vi "Constructor.vi"(8 "error in (no error)":errorcluster, 10 "Column Configuration":refnum<class "Basic Column Configuration.lvclass">, 11 "Column in":refnum<class "Column Parent.lvclass">) -> (0 "error out":errorcluster, 3 "Column out":refnum<class "Column Parent.lvclass">)   [LabVIEW 2020]
uses:
  Column Configuration/Basic Column Configuration Class/Basic Column Configuration.lvclass
  Column Parent.lvclass
  C:/Users/User/Desktop/Raman Program/Database OOP/source/Database OOP/Column Libraries/Basic Columns/Basic Columns/Column Class/Column Parent.lvclass
  C:/Users/User/Desktop/Raman Program/Database OOP/source/Database OOP/Column Libraries/Column Interface/Column Interface Class/Column Interface.lvclass
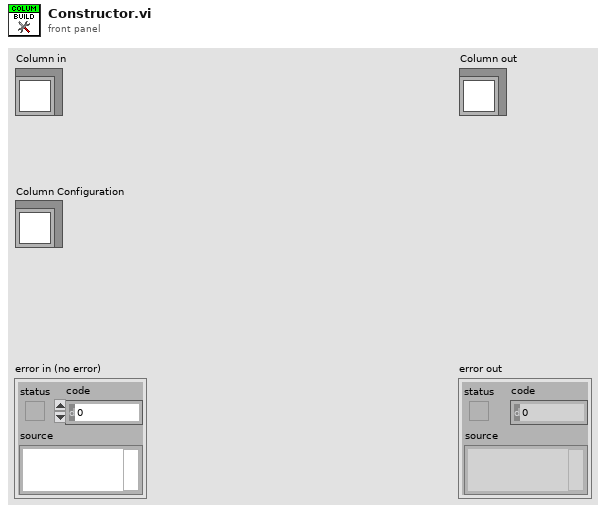
[diagram p1: front panel]
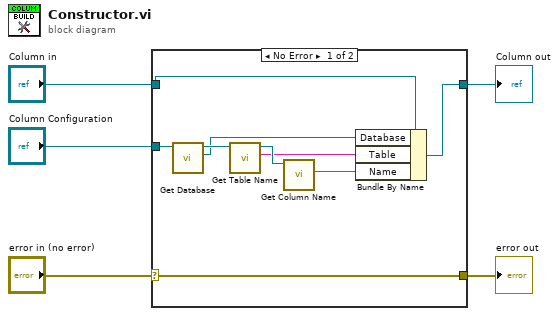
[diagram p0: block diagram]
diagram:
  n1 = case shown="No Error" "error in (no error)" {
    selector: "error in (no error)" -> [w6 w15]
    tunnel: [w6 w15] -> w5
    tunnel: "Column in" -> [w14 w16]
    tunnel: [w13 w16] -> w3
    tunnel: "Column Configuration" -> [w12 _]
    frame No Error {
      n2 = call-dynamic "Get Database.vi"("Basic Column Configuration in"=w12) -> ("Database"=w7:refnum<class "Database Interface.lvclass">, "Basic Column Configuration out"=w11:refnum<class "Basic Column Configuration.lvclass">)  [unwired: 8 in, 1 out]
      n3 = call-dynamic "Get Table Name.vi"("Basic Column Configuration in"=w11) -> ("Table Name"=w8:string, "Basic Column Configuration out"=w10:refnum<class "Basic Column Configuration.lvclass">)  [unwired: 8 in, 1 out]
      n4 = call-dynamic "Get Column Name.vi"("Basic Column Configuration in"=w10) -> ("Column Name"=w9:string)  [unwired: 8 in, 2 out]
      n5 = Bundle By Name(cluster=w14, "Database"=w7, "Table"=w8, "Name"=w9) -> (w13:refnum<class "Column Parent.lvclass">)
    }
    frame Error {
    }
  }
  "error out" <- w5
  "Column out" <- w3
